vi "CopyItem.vi"(5 "Max Column Count (10)":i32=10, 7 "Insert Inex":i32, 8 "error in (no error)":errorcluster, 9 "Parent Tag":string, 10 "Source Tag":string, 11 "TreeControl in":refnum<vi>) -> (0 "error out":errorcluster, 2 "Copied Tag":string, 3 "TreeControl out":refnum<vi>)   [LabVIEW 2020, in "TreeControlLib.lvlib"]
uses:
  TreeControlLib.lvlib
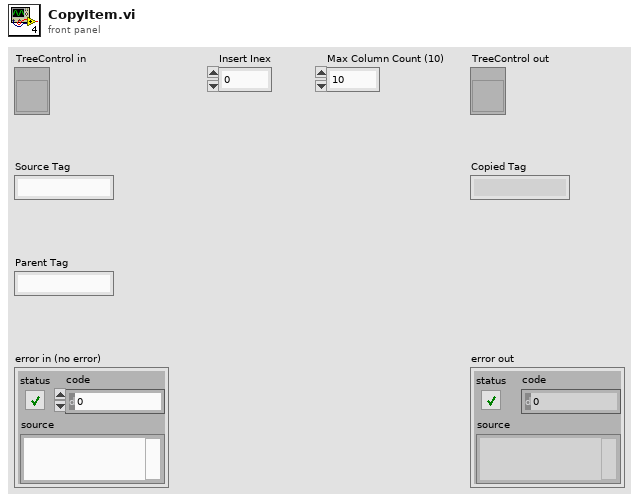
[diagram p1: front panel]
types:
  T1 = typedef "LVFontTypeDef.ctl" = cluster{"Font Name":string, "Size":u16, "Bold":bool, "Italic":bool, "Underline":bool, "Strikeout":bool, "Color":u32}
  T2 = typedef "LVBoundsTypeDef.ctl" = cluster{"Width":u32, "Height":u32}
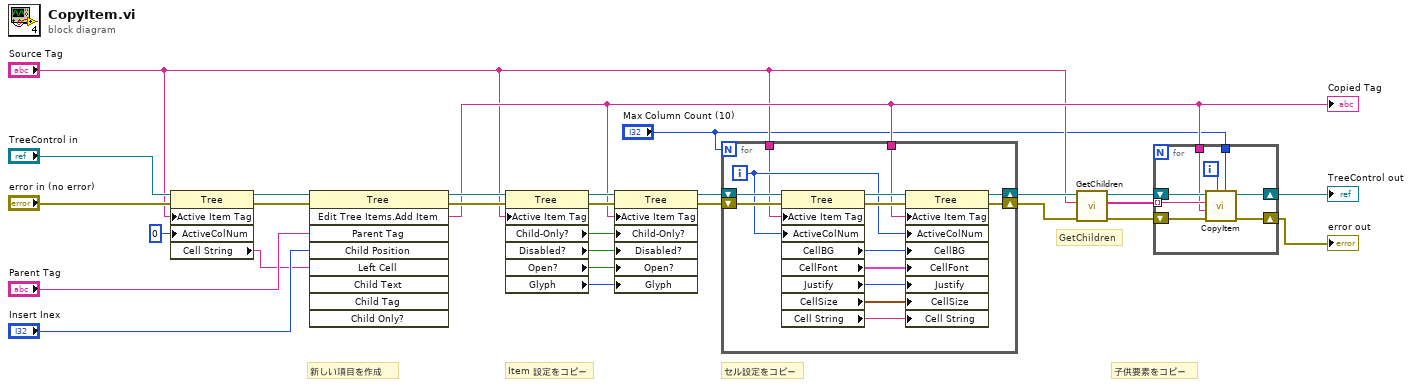
[diagram p0: block diagram]
diagram:
  # "子供要素をコピー"
  # "GetChildren"
  # "セル設定をコピー"
  # "Item 設定をコピー"
  # "新しい項目を作成"
  n1 = property class="Tree"(reference="TreeControl in", error in="error in (no error)", "Active Item Tag"="Source Tag", "ActiveColNum"=0 ("Active Cell:Active Column Number")) -> (reference out=w6:refnum<vi>, error out=w5:errorcluster, "Cell String"=w2:string)
  n2 = invoke class="Tree" method="Edit Tree Items.Add Item"(reference=w6, error in=w5, "Parent Tag"="Parent Tag", "Child Position"="Insert Inex", "Left Cell"=w2) -> (reference out=w26:refnum<vi>, error out=w25:errorcluster, "Edit Tree Items:Add Item"=w9:string)  [unwired: 4 in, 6 out]
  "Copied Tag" <- w9
  n3 = property class="Tree"(reference=w26, error in=w25, "Active Item Tag"="Source Tag") -> (reference out=w24:refnum<vi>, error out=w23:errorcluster, "Child-Only?"=w22:bool, "Disabled?"=w21:bool, "Open?"=w20:bool, "Glyph"=w19:i32)
  n4 = property class="Tree"(reference=w24, error in=w23, "Active Item Tag"=w9, "Child-Only?"=w22, "Disabled?"=w21, "Open?"=w20, "Glyph"=w19) -> (reference out=w18:refnum<vi>, error out=w17:errorcluster)
  n5 = for {
    N: "Max Column Count (10)" -> [_]
    tunnel: "Source Tag" -> [w32]
    tunnel: w9 -> [w31]
    shift-right: [w30] -> w16
    shift-left: w18 -> [w42]
    shift-right: [w29] -> w15
    shift-left: w17 -> [w41]
    i -> [w33]
    n6 = property class="Tree"(reference=w42, error in=w41, "Active Item Tag"=w32, "ActiveColNum"=w33) -> (reference out=w40:refnum<vi>, error out=w39:errorcluster, "CellBG"=w38:u32, "CellFont"=w37:T1, "Justify"=w36:enum16{"Left", "Center", "Right"}, "CellSize"=w35:T2, "Cell String"=w34:string)
    n7 = property class="Tree"(reference=w40, error in=w39, "Active Item Tag"=w31, "ActiveColNum"=w33, "CellBG"=w38, "CellFont"=w37, "Justify"=w36, "CellSize"=w35, "Cell String"=w34) -> (reference out=w30:refnum<vi>, error out=w29:errorcluster)
  }
  n8 = call "GetChildren.vi"("error in (no error)"=w15, "Parent Tag"="Source Tag", "TreeControl in"=w16) -> ("error out"=w13:errorcluster, "Children Tag"=w10:string[], "TreeControl out"=w14:refnum<vi>)  [unwired: 6 in]
  n9 = for {
    shift-right: [w47] -> w11
    shift-left: w14 -> [w50]
    shift-right: [w48] -> w12
    shift-left: w13 -> [w49]
    tunnel: w10 -> [w46] mode=indexing
    tunnel: w9 -> [w45]
    tunnel: "Max Column Count (10)" -> [w43]
    i -> [w44]
    n10 = call "CopyItem.vi"("Max Column Count (10)"=w43, "Insert Inex"=w44, "error in (no error)"=w49, "Parent Tag"=w45, "Source Tag"=w46, "TreeControl in"=w50) -> ("error out"=w48:errorcluster, "TreeControl out"=w47:refnum<vi>)  [unwired: 3 in, 1 out]
  }
  "TreeControl out" <- w11
  "error out" <- w12
